vi "Pre Launch Init.vi"(11 "CameraTestingUI in":refnum<class "CameraTestingUI.lvclass">) -> (0 "error out":errorcluster, 3 "CameraTestingUI out":refnum<class "CameraTestingUI.lvclass">)   [LabVIEW 2020, in "CameraTestingUI.lvlib" / "CameraTestingUI.lvclass"]
doc: "(<B>Filename</B>: Actor Framework.lvlib:Actor.lvclass:Pre Launch Init.vi)\n\nDefines behavior that occurs after the Launch Nested Actor method is invoked but before the actor's Actor Core method begins running.\n\nBy default, this method does nothing. A descendant class may override it to define behavior."
uses:
  CameraTestingUI.lvclass
  CameraTestingUI.lvclass/CameraTestingUI.ctl
  <vilib>/ActorFramework/Actor/Actor.lvclass
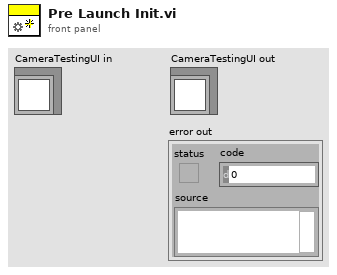
[diagram p1: front panel]
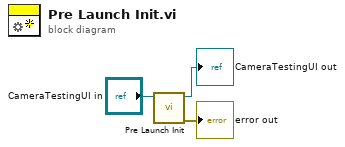
[diagram p0: block diagram]
diagram:
  n1 = call-parent "Pre Launch Init.vi"("Actor in"="CameraTestingUI in") -> ("error out"=→"error out":errorcluster, "Actor out"=→"CameraTestingUI out":refnum<class "CameraTestingUI.lvclass">)  [unwired: 9 in]
